vi "Channel Counts.vi"(8 "error in (no error)":errorcluster, 11 "VoiceMeeterRemote in":refnum<class "VoiceMeeterRemote.lvclass">) -> (0 "error out":errorcluster, 2 "Channel Counts":i32[](array[numeric]), 3 "VoiceMeeterRemote out":refnum<class "VoiceMeeterRemote.lvclass">)   [LabVIEW 2020, in "VoiceMeeterRemote.lvlib" / "VoiceMeeterRemote.lvclass"]
doc: "Returns the number of channels for each device index. For instance A1, index 0, has 2 audio channels whereas B1, index will vary based on the connected Voicemeeter type, has 8 audio channels."
uses:
  VoiceMeeterRemote.lvclass
  VoiceMeeterRemote.lvclass/VoiceMeeterRemote.ctl
  VoiceMeeterRemote.lvlib
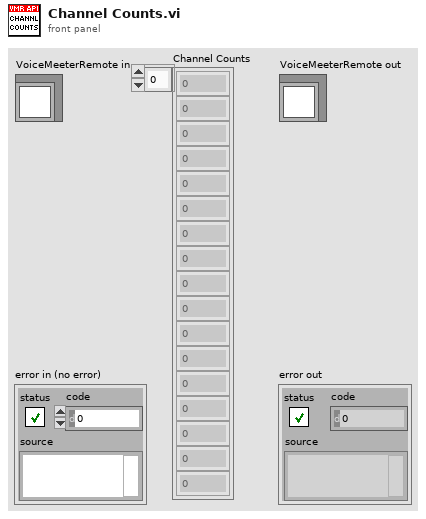
[diagram p1: front panel]
types:
  T1 = typedef "VoiceMeeterRemote.lvlib/Voicemeeter Type.ctl" = enum16{"Unknown", "Voicemeeter", "Banana", "Potato", "Potato x64"}
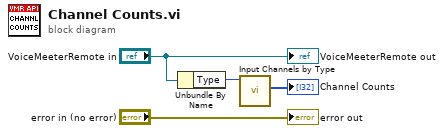
[diagram p0: block diagram]
diagram:
  n1 = Unbundle By Name("VoiceMeeterRemote in") -> ("Type"=w2:T1)
  n2 = call "Input Channels by Type.vi"("Voicemeeter Type"=w2) -> ("Channel Count"=→"Channel Counts":i32[])  [unwired: 10 in]
  "error out" <- "error in (no error)"
  "VoiceMeeterRemote out" <- "VoiceMeeterRemote in"
